vi "PWM Write.vi"(7 "PWM line":T1=1700 items=["Port0/DIO4 (Left Motor)"=1004, "Port0/DIO5 (Right Motor)"=1005, "Port0/DIO7 (Servo)"=1007, "Port7/DIO0"=1700, "Port7/DIO1"=1701, "Port7/DIO2"=1702, "Port7/DIO3"=1703], 8 "error in (no error)":errorcluster, 9 "pulse width (us)":u32=1500, 10 "period (us)":u32=20000, 11 "direct IO in":refnum<class "NI_Robotics_Starter Kit Direct IO_FPGA.lvclass">) -> (0 "error out":errorcluster, 3 "direct IO out":refnum<class "NI_Robotics_Starter Kit Direct IO_FPGA.lvclass">)   [LabVIEW 2017, in "NI_Robotics_Starter Kit Direct IO_FPGA.lvclass"]
uses:
  <vilib>/robotics/Starter Kit/FPGA Direct IO/NI_Robotics_Starter Kit Direct IO_FPGA.lvclass
  <vilib>/robotics/Starter Kit/Direct IO/PWM Lines.ctl
  <vilib>/robotics/Starter Kit/FPGA Direct IO/NI_Robotics_Starter Kit Direct IO_FPGA.lvclass/NI_Robotics_Starter Kit Direct IO_FPGA.ctl
  <vilib>/rvi/errors/niLvFpgaAdjustHostInterfaceError.vi
  <vilib>/Utility/error.llb/Error Cluster From Error Code.vi
  <vilib>/robotics/Starter Kit/FPGA Direct IO/Direct IO FPGA Ref.ctl
  <vilib>/rvi/interface/nirviReadWriteControl/nirviReadWriteControl.xnode
  NiFpgaLv.dll
  <vilib>/rvi/interface/Simulation/niFpgaSimulationCallBeginRW.vi
  <vilib>/robotics/Starter Kit/Direct IO/NI_Robotics_Starter Kit Direct IO.lvclass
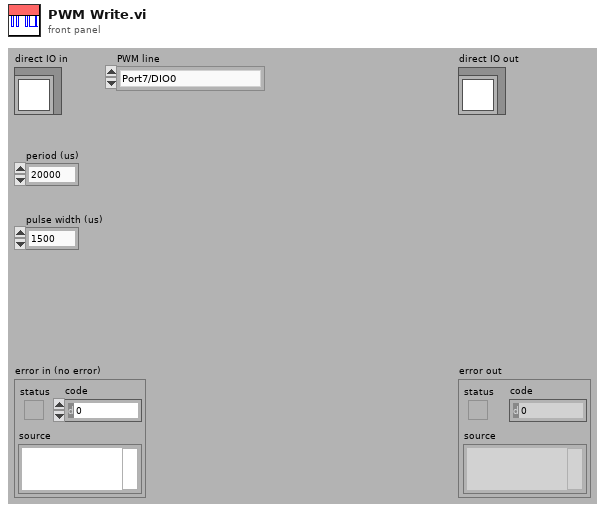
[diagram p1: front panel]
types:
  T1 = typedef "NI_Robotics_Starter Kit Direct IO.lvclass/PWM Lines.ctl" = u16
  T2 = cluster{"period (us)":u32, "pulse width (us)":u32}
  T3 = typedef "NI_Robotics_Starter Kit Direct IO_FPGA.lvclass/Direct IO FPGA Ref.ctl" = refnum<k20>
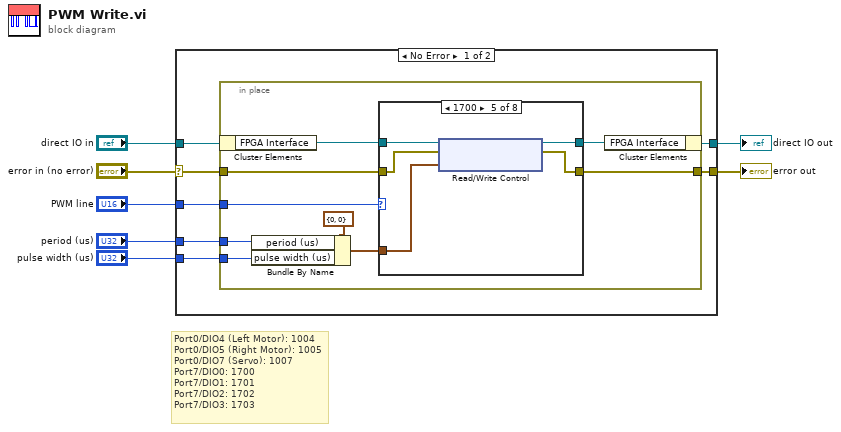
[diagram p0: block diagram]
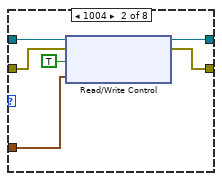
[diagram p3: hidden frame]
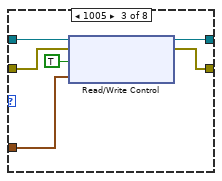
[diagram p4: hidden frame]
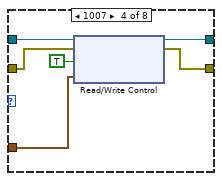
[diagram p5: hidden frame]
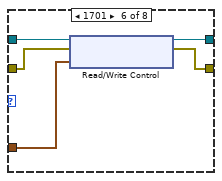
[diagram p6: hidden frame]
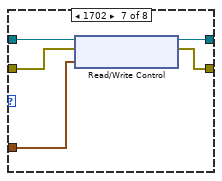
[diagram p7: hidden frame]
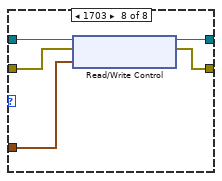
[diagram p8: hidden frame]
diagram:
  # "Port0/DIO4 (Left Motor): 1004\nPort0/DIO5 (Right Motor): 1005\nPort0/DIO7 (Servo): 1007\nPort7/DIO0: 1700\nPort7/DIO1: 1701\nPort7/DIO2: 1702\nPort7/DIO3: 1703"
  n1 = case shown="No Error" "error in (no error)" {
    selector: "error in (no error)" -> [w12 w65]
    tunnel: [w11 w65] -> w4
    tunnel: "direct IO in" -> [w14 w64]
    tunnel: [w10 w64] -> w5
    tunnel: "PWM line" -> [w13 _]
    tunnel: "period (us)" -> [w9 _]
    tunnel: "pulse width (us)" -> [w8 _]
    frame No Error {
      n2 = in-place {
        in-place-border: w13 -> [w23]
        in-place-border: w12 -> [w21]
        in-place-border: [w19] -> w11
        in-place-border: w9 -> [w16]
        in-place-border: w8 -> [w15]
        n3 = in-place-cluster #1(w14) -> ("FPGA Interface"=w22:T3)
        n4 = Bundle By Name(cluster=T2 {"period (us)"=0, "pulse width (us)"=0} ("PWM_0"), "period (us)"=w16, "pulse width (us)"=w15) -> (w17:T2)
        n5 = case shown="1700" w23 {
          tunnel: w22 -> [w25 w31 w37 w43 w48 w53 w58 w63]
          tunnel: w21 -> [w24 w29 w35 w41 w46 w50 w55 w60]
          tunnel: [w25 w30 w36 w42 w47 w52 w57 w62] -> w20
          tunnel: [w24 w28 w34 w40 w45 w51 w56 w61] -> w19
          tunnel: w17 -> [_ w26 w32 w38 w44 w49 w54 w59]
          frame Default {
          }
          frame 1004 {
            n6 = xnode "Read/Write Control"("FPGA VI Reference In"=w31, "error in"=w29, "DCmotor_0_direct"=TRUE, "DCmotor_0_PWM"=w26) -> ("FPGA VI Reference Out"=w30:T3, "error out"=w28:errorcluster)
          }
          frame 1005 {
            n7 = xnode "Read/Write Control"("FPGA VI Reference In"=w37, "error in"=w35, "DCmotor_1_direct"=TRUE, "DCmotor_1_PWM"=w32) -> ("FPGA VI Reference Out"=w36:T3, "error out"=w34:errorcluster)
          }
          frame 1007 {
            n8 = xnode "Read/Write Control"("FPGA VI Reference In"=w43, "error in"=w41, "servo_0_direct"=TRUE, "servo_0_PWM"=w38) -> ("FPGA VI Reference Out"=w42:T3, "error out"=w40:errorcluster)
          }
          frame 1700 {
            n9 = xnode "Read/Write Control"("FPGA VI Reference In"=w48, "error in"=w46, "Port7/DIO0_PWM"=w44) -> ("FPGA VI Reference Out"=w47:T3, "error out"=w45:errorcluster)
          }
          frame 1701 {
            n10 = xnode "Read/Write Control"("FPGA VI Reference In"=w53, "error in"=w50, "Port7/DIO1_PWM"=w49) -> ("FPGA VI Reference Out"=w52:T3, "error out"=w51:errorcluster)
          }
          frame 1702 {
            n11 = xnode "Read/Write Control"("FPGA VI Reference In"=w58, "error in"=w55, "Port7/DIO2_PWM"=w54) -> ("FPGA VI Reference Out"=w57:T3, "error out"=w56:errorcluster)
          }
          frame 1703 {
            n12 = xnode "Read/Write Control"("FPGA VI Reference In"=w63, "error in"=w60, "Port7/DIO3_PWM"=w59) -> ("FPGA VI Reference Out"=w62:T3, "error out"=w61:errorcluster)
          }
        }
        n13 = in-place-cluster #1("FPGA Interface"=w20) -> (w10:refnum<class "NI_Robotics_Starter Kit Direct IO_FPGA.lvclass">)
      }
    }
    frame Error {
    }
  }
  "error out" <- w4
  "direct IO out" <- w5
